vi "Form_mode_name.vi"(1 "Params":string[](array[string]), 2 "Mode_name_in":string) -> (0 "Mode name out":string)   [LabVIEW 2020]
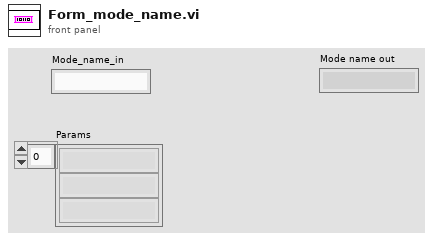
[diagram p1: front panel]
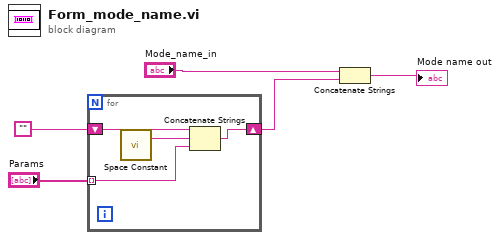
[diagram p0: block diagram]
diagram:
  n1 = for {
    tunnel: "Params" -> [w9] mode=indexing
    shift-right: [w7] -> w2
    shift-left: "" -> [w8]
    n2 = call <vilib>:"Space Constant.vi"() -> ("String"=w6:string)
    n3 = Concatenate Strings(w8, w6, w9) -> (w7:string)
  }
  n4 = Concatenate Strings("Mode_name_in", w2) -> (→"Mode name out":string)
